vi "Bertta_v09_61.vi"() -> ()   [LabVIEW 2015]
uses:
  x64/Debug/BERTTA.dll
panel:
  out "element":bool
  out "Started:":string
  in  "SHUTDOWN":bool
  in  "MASTER CONTROL":bool
  in  "Tab Control":T1(tab)
  in  "Read Seq":bool
  in  "Save Seq":bool
  in  "Configuration file":path=path "C:/Users/shresplab/Desktop/BerttaConfiguration.lvm" caption="Filename"
  in  "OK Button 2":bool
  out "Boolean":bool
  in  "User (initials)":string
  in  "Project name":string
  in  "Description":string
  out "Output file":string
  out "PUMP1":bool
  out "Target amount":dbl
  out "Scale weight":dbl
  out "Amount now":dbl
  out "Flow rate":dbl
  out "Time to target":dbl format="%<%H:%M:%S>t"
  out "Current step":dbl
  out "Target":dbl
  out "Amount now":dbl
  out "Amount now":dbl
  out "Target":dbl
  out "Current step":dbl
  out "Time to target":dbl format="%<%H:%M:%S>t"
  out "Flow rate":dbl
  out "Amount now":dbl
  out "Scale weight":dbl
  out "Target amount":dbl
  out "PUMP2":bool
  out "Sensor OK 6":bool
  out "Sensor OK 5":bool
  out "Sensor OK 4":bool
  out "Sensor OK 3":bool
  in  "OK Button":bool
  in  "Add comment":string
  out "PUMP3":bool
  out "Target amount":dbl
  out "Scale weight":dbl
  out "Amount now":dbl
  out "Flow rate":dbl
  out "Time to target":dbl format="%<%H:%M:%S>t"
  out "Current step":dbl
  out "Target":dbl
  out "Amount now":dbl
  out "Tr":dbl
  out "Tj in":dbl
  out "Tj out":dbl
  out "T set":dbl
  out "Current step":i32
  out "RPM":dbl
  out "Torque 2":dbl
  out "Waveform Chart 5":dynamicdata(graph)
  out "Waveform Chart 6":dynamicdata(graph)
  out "Waveform Chart 7":dynamicdata(graph)
  in  "Tab Control 2":T2(tab)
  out "Waveform Chart 3":dynamicdata(graph)
  out "Waveform Chart 8":dynamicdata(graph)
  out "Waveform Chart 11":dynamicdata(graph)
  out "Waveform Chart 13":dynamicdata(graph)
  out "Waveform Chart 9":dynamicdata(graph)
  out "Table":string[][](table)=[["14.8.2017 18.06.59", "0,000000", "417,670000", "-0,150000", "1,000000", "22,220000", "23,366837", "23,574959", "23,985852", "23,690000", "240,000000", "4,000000", "0,000000", "397,000000", "-397,000000", "1,000000"], ["14.8.2017 18.07.06", "0,000000", "417,640000", "-0,120000", "1,000000", "22,220000", "23,763115", "23,906257", "23,985694", "23,680000", "240,000000", "4,000000", "0,000000", "397,000000", "-397,000000", "1,000000"], ["14.8.2017 18.07.13", "0,000000", "417,640000", "-0,120000", "1,000000", "22,220000", "23,965922", "24,013440", "23,984906", "23,670000", "240,000000", "4,100000", "3,000000", "397,000000", "-397,000000", "1,000000"], ["14.8.2017 18.07.21", "0,000000", "417,640000", "-0,120000", "1,000000", "22,220000", "23,943860", "23,900110", "23,987113", "23,670000", "240,000000", "4,000000", "0,000000", "397,000000", "-397,000000", "1,000000"], ["14.8.2017 18.07.28", "0,000000", "417,640000", "-0,120000", "1,000000", "22,220000", "23,736328", "23,600018", "23,989004", "23,660000", "240,000000", "4,000000", "0,000000", "397,000000", "-397,000000", "1,000000"], ["14.8.2017 18.07.36", "0,000000", "417,640000", "-0,120000", "1,000000", "22,220000", "23,480910", "23,324538", "23,991053", "23,660000", "240,000000", "4,000000", "0,000000", "397,000000", "-397,000000", "1,000000"], ["14.8.2017 18.07.43", "0,000000", "417,640000", "-0,120000", "2,000000", "22,220000", "23,195579", "23,008270", "23,999093", "23,650000", "240,000000", "4,000000", "0,000000", "397,000000", "-397,000000", "1,000000"], ["14.8.2017 18.07.51", "0,000000", "417,650000", "-417,650000", "1,000000", "22,220000", "22,862541", "22,649021", "24,003979", "23,650000", "240,000000", "4,000000", "0,000000", "397,000000", "-397,000000", "2,000000"], ["14.8.2017 18.07.58", "0,000000", "417,640000", "0,010000", "1,000000", "22,220000", "22,541353", "22,354878", "24,005398", "23,650000", "240,000000", "4,000000", "0,000000", "397,000000", "-397,000000", "1,000000"], ["14.8.2017 18.08.06", "0,000000", "417,640000", "0,010000", "1,000000", "22,220000", "22,347931", "22,253738", "24,007605", "23,640000", "240,000000", "4,100000", "0,000000", "397,000000", "-397,000000", "1,000000"], ["14.8.2017 18.08.13", "0,000000", "417,640000", "0,010000", "1,000000", "22,220000", "22,329030", "22,302102", "24,006028", "23,640000", "240,000000", "4,000000", "0,000000", "395,820000", "-395,820000", "1,000000"], ["14.8.2017 18.08.20", "0,000000", "417,640000", "0,010000", "1,000000", "22,220000", "22,466849", "22,511320", "24,002403", "23,630000", "240,000000", "4,000000", "0,000000", "395,830000", "-0,010000", "1,000000"], ["14.8.2017 18.08.28", "0,000000", "417,640000", "0,010000", "1,000000", "22,220000", "22,707062", "22,835101", "24,000984", "23,620000", "240,000000", "4,000000", "0,000000", "395,830000", "-0,010000", "1,000000"], ["14.8.2017 18.08.35", "0,000000", "417,640000", "0,010000", "1,000000", "22,220000", "23,054104", "23,232979", "24,001299", "23,600000", "240,000000", "4,000000", "0,000000", "395,830000", "-0,010000", "1,000000"], ["14.8.2017 18.08.43", "0,000000", "417,640000", "0,010000", "1,000000", "22,220000", "23,412371", "23,522793", "24,002560", "23,590000", "240,000000", "4,000000", "0,000000", "395,820000", "0,000000", "1,000000"], ["14.8.2017 18.08.51", "0,000000", "417,640000", "0,010000", "1,000000", "22,220000", "23,596247", "23,656125", "24,003821", "23,580000", "240,000000", "4,000000", "0,000000", "395,820000", "0,000000", "1,000000"]]
  in  "Reset":bool
  in  "Numeric 4":dbl=20.0
  in  "Numeric 3":dbl=30.0
  in  "Numeric 2":dbl=40.0
  in  "Numeric 1":dbl=30.0
  in  "Numeric":dbl=20.0
  out "Boolean 12":bool
  out "Boolean 7":bool
  out "Boolean 6":bool
  out "Boolean 5":bool
  out "Boolean 4":bool
  out "Boolean 19":bool
  in  "Numeric 5":dbl=5.0
  in  "Numeric 6":dbl=5.0
  in  "Numeric 7":dbl=5.0
  in  "Numeric 8":dbl=5.0
  in  "T ext / T ext 2":enum32{"External 1", "External 2"}(radio)
  out "Sensor OK":bool
  in  "T fail":dbl=20.0
  in  "?":bool
  in  "T manual setpoint":dbl=20.0
  in  "Lauda port":dbl=9.0
  in  "Manual select":enum32{"Tr", "Tj"}(radio)
  in  "PAUSE":bool
  out "Waveform Chart":dynamicdata(graph)
  out "T external 2":dbl
  out "Led11 5":bool
  in  "Port":i32=10
  in  "Radio Buttons 4":enum32{"Reglo Digital", "Reglo Analog", "PAM"}(radio)
  out "Speed":dbl
  out "mA":dbl format="%#_2g"
  in  "Port":i32=16
  out "RPM":dbl format="%_4f"
  out "Led10 3":bool
  out "Led9 3":bool
  out "Led8 3":bool
  out "Led7 3":bool
  out "Led6 3":bool
  out "Led5 3":bool
  out "Led4 3":bool
  out "Led3 3":bool
  out "Led2 3":bool
  out "Led1 3":bool
  in  "PumpSeq 4":dbl[][](array[numeric])=[[1.0, 1.0, 7.0], [2.0, 1.0, 2.0], [3.0, 1.0, 100.0], [0.0, 0.0, 0.0], [0.0, 0.0, 0.0], [0.0, 0.0, 0.0], [0.0, 0.0, 0.0], [0.0, 0.0, 0.0], [0.0, 0.0, 0.0], [0.0, 0.0, 0.0], [0.0, 1.0, 0.0]]
  in  "?":bool
  out "Flow rate (g/min)":dbl
  out "Scale reading":dbl
  out "Step amount now":dbl
  in  "Grams / min":dbl
  out "Waveform Chart 14":dynamicdata(graph)
  in  "?":bool
  out "Total amount now":dbl
  out "Total time 4":dbl
  out "Total amount target 4":dbl
  out "Led11 4":bool
  in  "Reset 5":bool
  out "Elapsed / step":i32
  out "Time to target":dbl format="%<%H:%M:%S>t"
  out "Led11":bool
  in  "Port":i32=11
  in  "Radio Buttons 2":enum32{"Reglo Digital", "Reglo Analog", "PAM"}(radio)
  out "Speed":dbl
  out "mA":dbl format="%#_2g"
  in  "Port":i32=15
  out "RPM":dbl format="%_4f"
  out "Led10":bool
  out "Led9":bool
  out "Led8":bool
  out "Led7":bool
  out "Led6":bool
  out "Led5":bool
  out "Led4":bool
  out "Led3":bool
  out "Led2":bool
  out "Led1":bool
  in  "PumpSeq 2":dbl[][](array[numeric])=[[1.0, 1.0, 7.0], [2.0, 1.0, 2.0], [3.0, 1.0, 100.0], [0.0, 0.0, 0.0], [0.0, 0.0, 0.0], [0.0, 0.0, 0.0], [0.0, 0.0, 0.0], [0.0, 0.0, 0.0], [0.0, 0.0, 0.0], [0.0, 0.0, 0.0], [0.0, 1.0, 0.0]]
  in  "?":bool
  out "Flow rate (g/min)":dbl
  out "Scale reading":dbl
  out "Step amount now":dbl
  in  "Grams / min":dbl
  out "Waveform Chart 10":dynamicdata(graph)
  in  "?":bool
  out "Total amount now":dbl
  out "Total time 2":dbl
  out "Total amount target 2":dbl
  out "Led11":bool
  in  "Reset 3":bool
  out "Elapsed / step":i32
  out "Time to target":dbl format="%<%H:%M:%S>t"
  out "Led11 3":bool
  in  "Port":i32=12
  in  "Radio Buttons 3":enum32{"Reglo Digital", "Reglo Analog", "PAM"}(radio)
  out "Speed":dbl
  out "mA":dbl format="%#_2g"
  in  "Port":i32=14
  out "RPM":dbl format="%_4f"
  out "Led10 2":bool
  out "Led9 2":bool
  out "Led8 2":bool
  out "Led7 2":bool
  out "Led6 2":bool
  out "Led5 2":bool
  out "Led4 2":bool
  out "Led3 2":bool
  out "Led2 2":bool
  out "Led1 2":bool
  in  "PumpSeq 3":dbl[][](array[numeric])=[[1.0, 1.0, 7.0], [2.0, 1.0, 2.0], [3.0, 1.0, 100.0], [0.0, 0.0, 0.0], [0.0, 0.0, 0.0], [0.0, 0.0, 0.0], [0.0, 0.0, 0.0], [0.0, 0.0, 0.0], [0.0, 0.0, 0.0], [0.0, 0.0, 0.0], [0.0, 1.0, 0.0]]
  in  "?":bool
  out "Flow rate (g/min)":dbl
  out "Scale reading":dbl
  out "Step amount now":dbl
  in  "Grams / min":dbl
  out "Waveform Chart 12":dynamicdata(graph)
  in  "?":bool
  out "Total amount now":dbl
  out "Total time 3":dbl
  out "Total amount target 3":dbl
  out "Led11 2":bool
  in  "Reset 4":bool
  out "Elapsed / step":i32
  out "Time to target":dbl format="%<%H:%M:%S>t"
  in  "Bypass select 2":enum32{"Remote", "Manual"}(radio)=enum."Manual"
  in  "Port":dbl=13.0
  out "RPM":dbl
  out "Torque":dbl
  in  "Set RPM":dbl(slide) scale=0.0..2000.0
  out "Waveform Chart 4":dynamicdata(graph)
  in  "Treshold (T/C)":dbl=0.5
  out "DAQ 9217 (PT100)":errorcluster
  # "Temperature sensor:"
  # "Manual control:"
  # "PUMP & SCALE 1"
  # "STEP"
  # "TOTAL"
  # "PUMP & SCALE 2"
  # "STEP"
  # "TOTAL"
  # "PUMP & SCALE 3"
  # "STEP"
  # "TOTAL"
  # "Manual control"
  # "Secondary temperature sensor"
  # "Device communication"
  # "Temp"
  # "Time"
  # "Grams    /   min"
  # "End of sequence"
  # "Manual control"
  # "Device communication"
  # "Pump configuration"
  # "Scale configuration"
  # "SCALE 1"
  # "Grams    /   min"
  # "End of sequence"
  # "Manual control"
  # "Device communication"
  # "Pump configuration"
  # "Scale configuration"
  # "SCALE 2"
  # "Grams    /   min"
  # "End of sequence"
  # "Manual control"
  # "Device communication"
  # "Pump configuration"
  # "Scale configuration"
  # "SCALE 3"
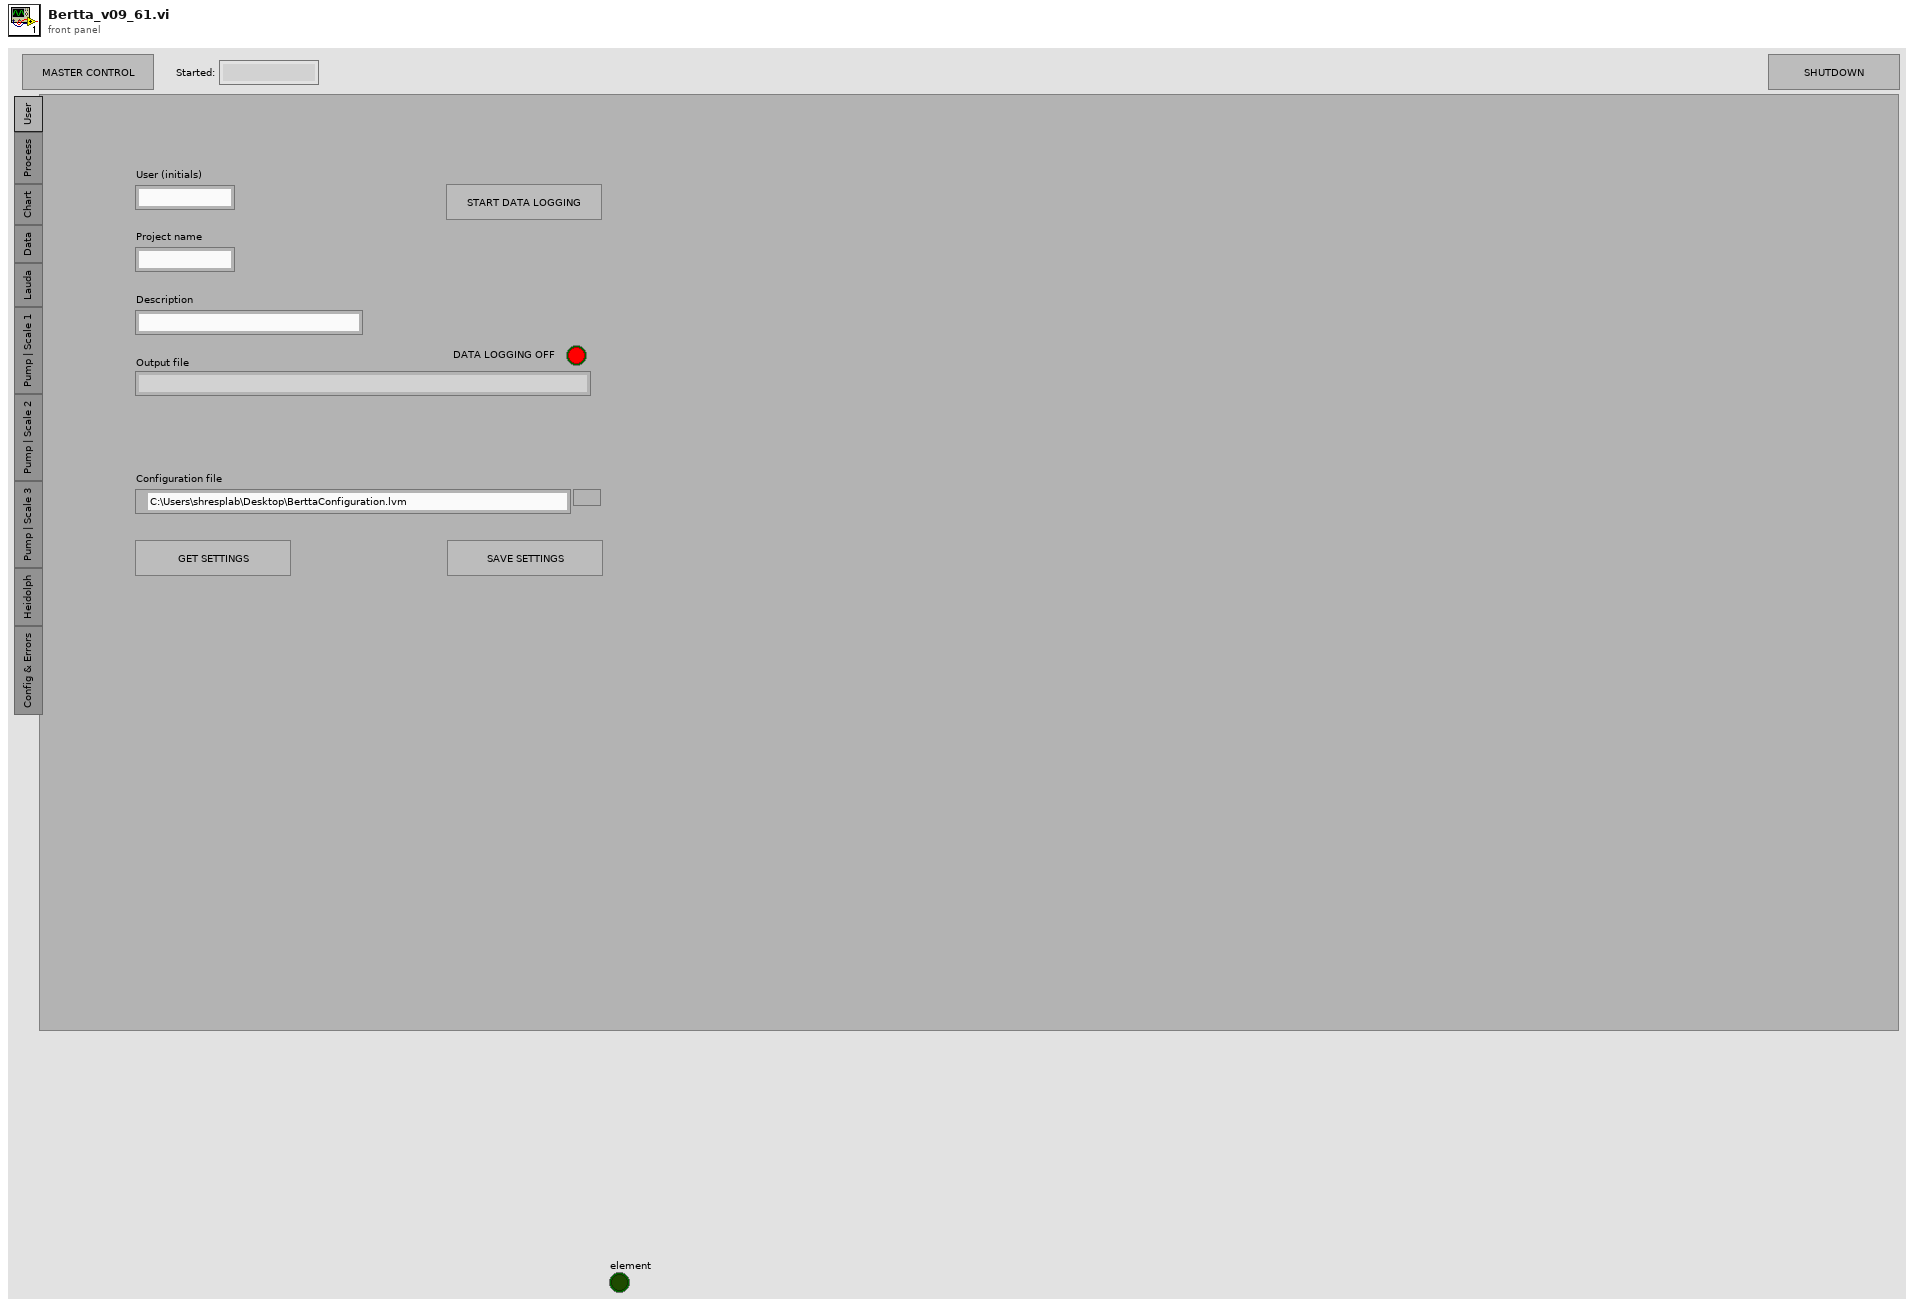
[diagram p1: front panel]
types:
  T1 = enum32{"User", "Process", "Chart", "Data", "Lauda", "Pump | Scale 1", "Pump | Scale 2", "Pump | Scale 3", "Heidolph", "Config & Errors"}
  T2 = enum32{"Temperatures", "Scale / Pump 1", "Scale / Pump 2", "Scale / Pump 3", "RPM / torque"}
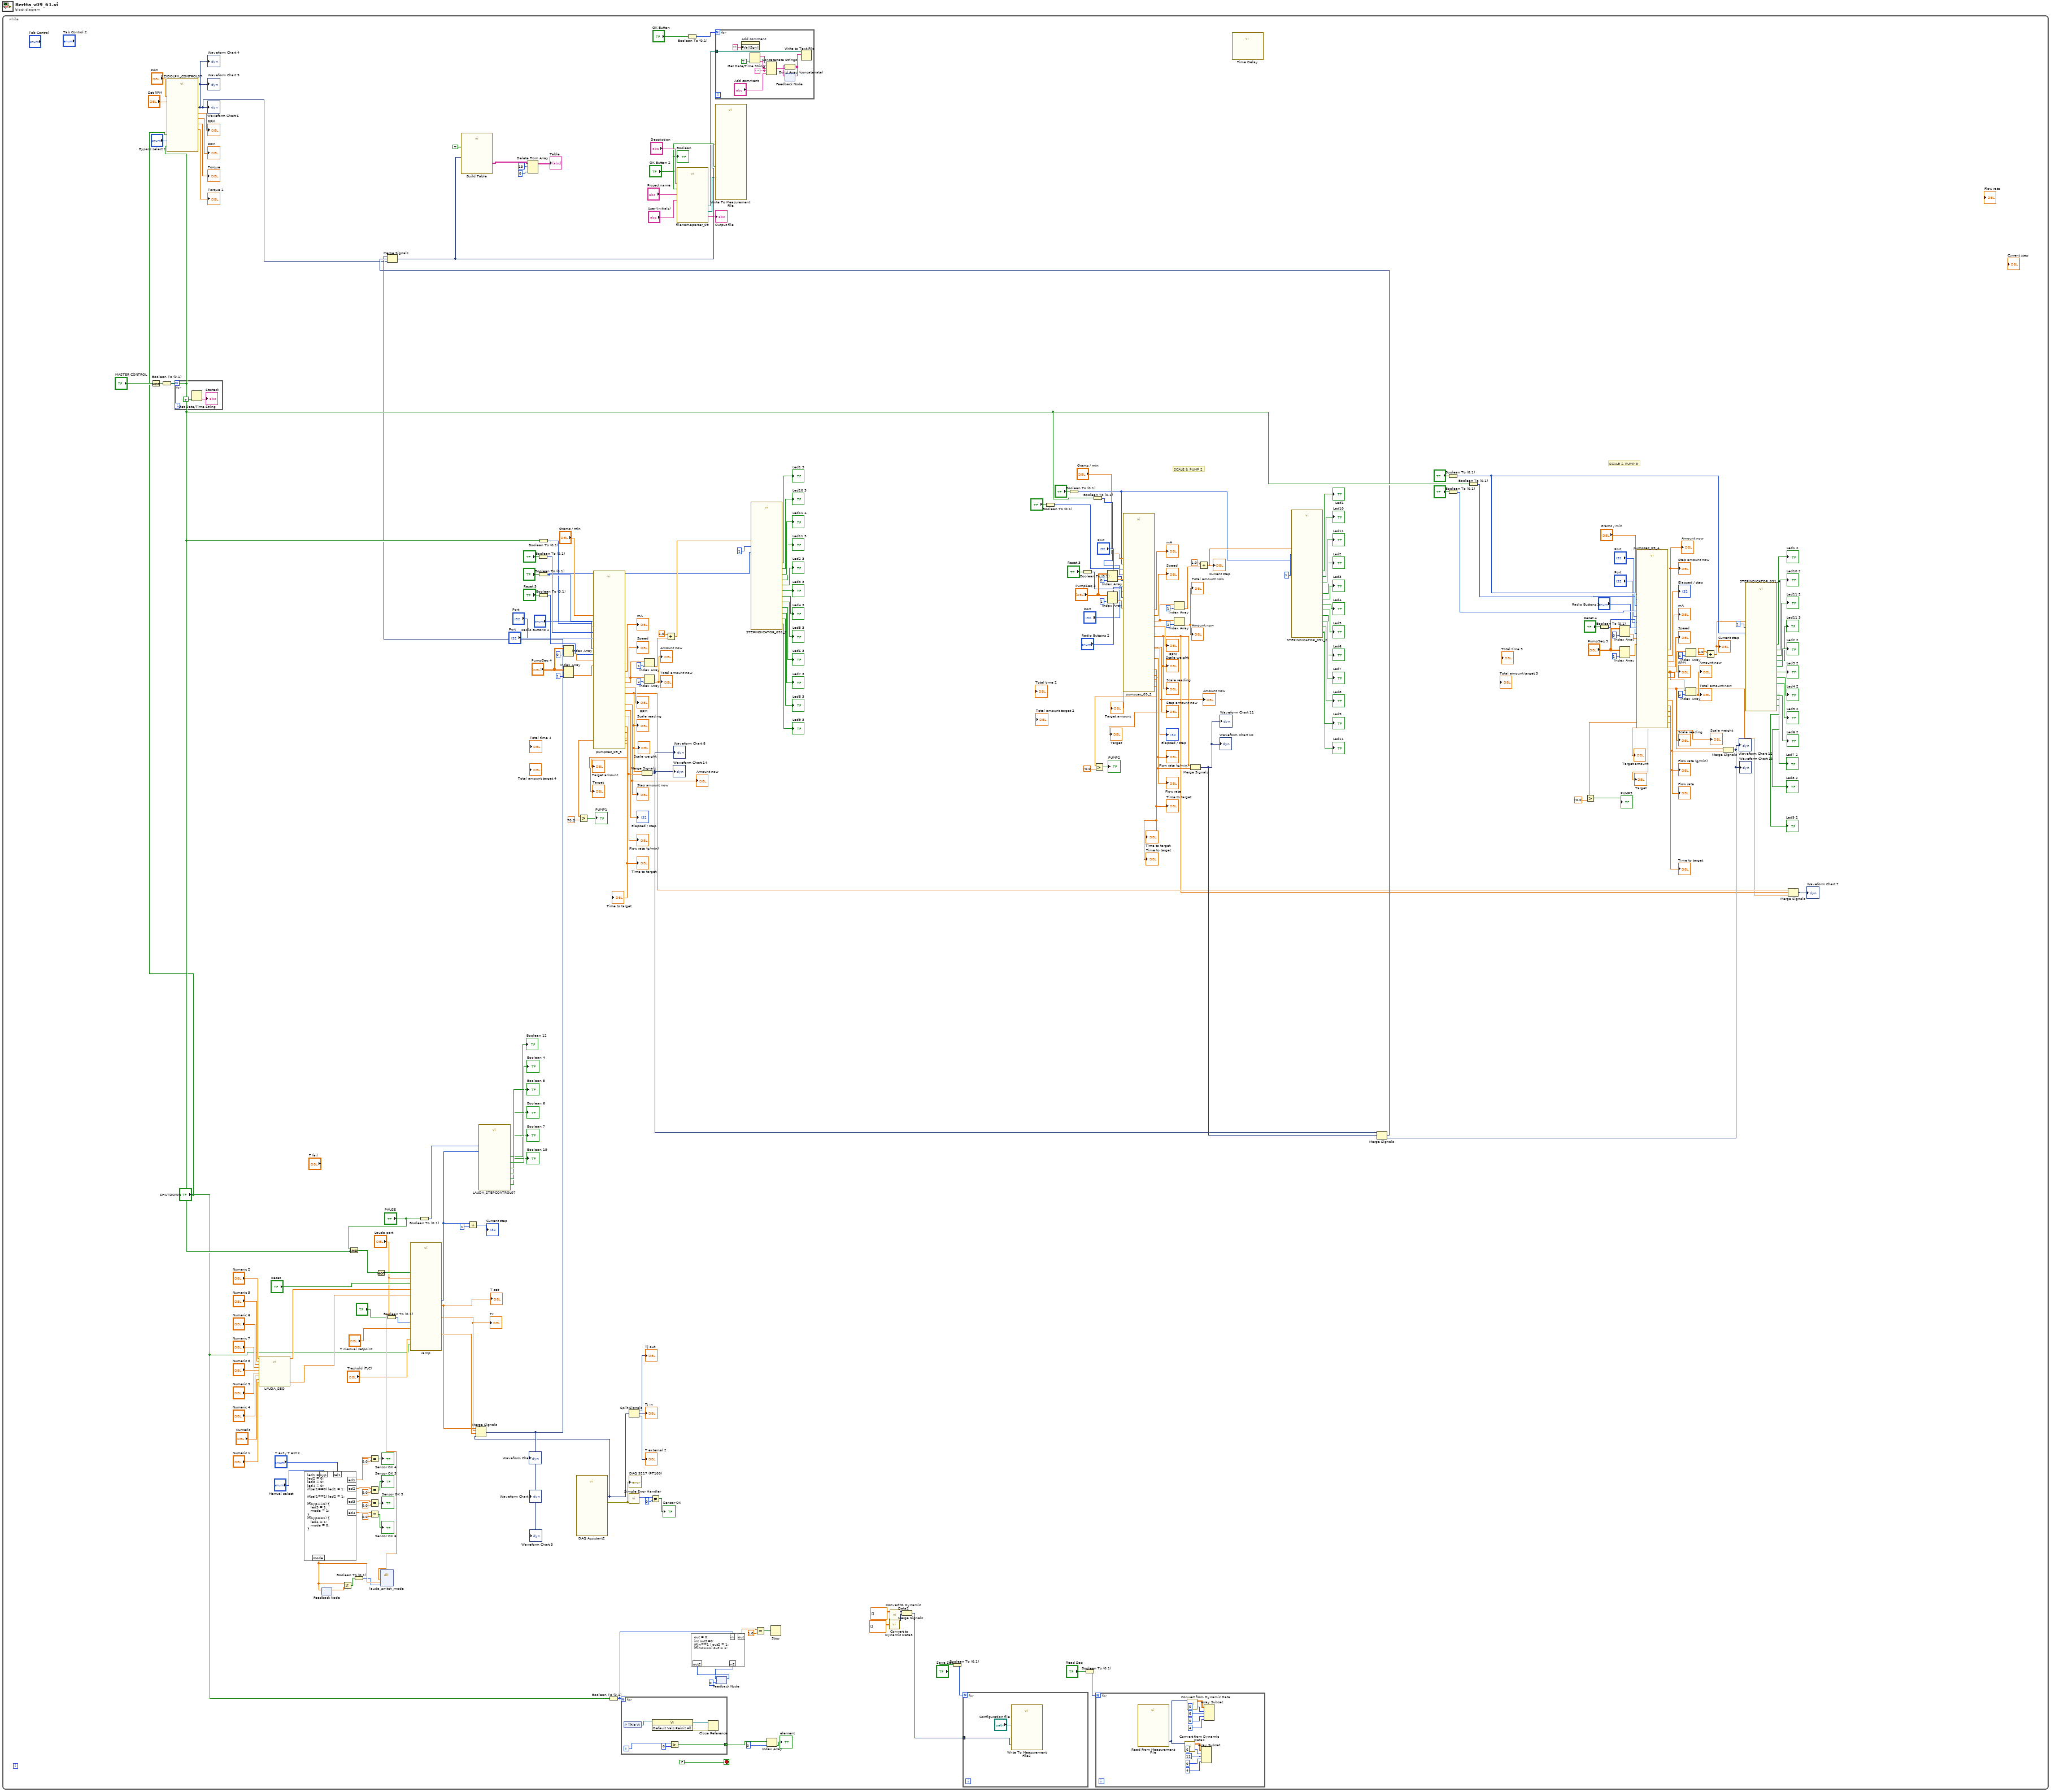
[diagram p0: block diagram]
diagram:
  n1 = while {
    stop <- FALSE stop-if-true
    # "SCALE & PUMP 3"
    # "SCALE & PUMP 2"
    n2 = Not(x="MASTER CONTROL") -> (.not. x?=w239:bool)
    n3 = Boolean To (0,1)(Boolean=w239) -> (0, 1=w240:i16)
    n4 = call "HEIDOLPH_CONTROL07.vi"("master"="MASTER CONTROL", "shutdown"="SHUTDOWN", "Bypass select"="Bypass select 2", "Set RPM"="Set RPM", "Device port"="Port") -> ("Dynamic Data"=w37:dynamicdata, "RPM"=→"RPM":dbl, "RPM 2"=→"RPM":dbl, "Torque"=→"Torque":dbl, "Torque 2"=→"Torque 2":dbl)  [unwired: 2 in]
    "Waveform Chart 4" <- w37
    "Waveform Chart 6" <- w37
    "Waveform Chart 9" <- w37
    n5 = for {
      N: w240 -> [_]
      n6 = Get Date/Time String(want seconds? (F)=TRUE) -> (time string=→"Started:":string)  [unwired: 2 in, 1 out]
    }
    n7 = call "LAUDA_SEQ.vi"("Numeric 2"="Numeric 2", "Numeric 1"="Numeric 1", "Numeric"="Numeric", "Numeric 5"="Numeric 5", "Numeric 6"="Numeric 6", "Numeric 7"="Numeric 7", "Numeric 8"="Numeric 8", "Numeric 3"="Numeric 3", "Numeric 4"="Numeric 4") -> ("output array"=w140:dbl[], "output array 2"=w139:dbl[])  [unwired: 5 in]
    n8 = formula code="led1 = 0;\nled2 = 0;\nled3 = 0;\nled4 = 0;\nif(sel1==0) led1 = 1;\n\nif(sel1==1) led2 = 1;\n\nif(byp==0) {\n   led3 = 1;\n   mode = 1;\n}\nif(byp==1) {\n   led4 = 1;\n   mode = 0;\n}"("sel1"="T ext / T ext 2", "byp"="Manual select") -> ("led1"=w209:dbl, "led2"=w207:dbl, "led3"=w202:dbl, "led4"=w201:dbl, "mode"=w134:dbl)
    n9 = feedback-in #1(w134) -> ()
    n10 = feedback #1() -> (w133:dbl)  [unwired: 1 in]
    n11 = Not Equal?(x=w134, y=w133) -> (x != y?=w131:bool)
    n12 = And(x="PAUSE", y="MASTER CONTROL") -> (x .and. y?=w152:bool)
    n13 = Boolean To (0,1)(Boolean=w131) -> (0, 1=w132:i16)
    n14 = Equal?(x=w209, y=0.0) -> (x = y?=→"Sensor OK 4":bool)
    n15 = Equal?(x=w207, y=0.0) -> (x = y?=→"Sensor OK 3":bool)
    n16 = Equal?(x=w202, y=0.0) -> (x = y?=→"Sensor OK 5":bool)
    n17 = Equal?(x=w201, y=0.0) -> (x = y?=→"Sensor OK 6":bool)
    n18 = Not(x=w152) -> (.not. x?=w151:bool)
    n19 = dll-call lib="C:/Users/shresplab/OneDrive - Kemira Oyj/Documents/Visual Studio 2017/Projects/Bertta/BERTTA/x64/Debug/BERTTA.dll" fn="lauda_switch_mode"("port"="Lauda port", "mode"=w134, "enable"=w132) -> ()  [unwired: 7 in, 2 out]
    n20 = Boolean To (0,1)(Boolean="?") -> (0, 1=w137:i16)
    n21 = call "ramp.vi"("pause"=w151, "manual"=w137, "T_man"="T manual setpoint", "Seq"=w140, "reset"="Reset", "TimeParams"=w139, "shutdown"="SHUTDOWN", "port"="Lauda port", "treshold"="Treshold (T/C)") -> ("T in"=w36:dbl, "STEP"=w3:i32, "T ext"=w21:dbl, "T control"=w22:dbl)  [unwired: 2 in, 1 out]
    "Tr" <- w21
    "T set" <- w22
    n22 = Boolean To (0,1)(Boolean="PAUSE") -> (0, 1=w196:i16)
    n23 = Add(x=w3, y=1) -> (x+y=→"Current step":i32)
    n24 = call "LAUDA_STEPCONTROL07.vi"("step"=w3, "pause"=w196) -> ("Boolean 13"=→"Boolean 19":bool, "Boolean 6"=→"Boolean 6":bool, "Boolean 5"=→"Boolean 5":bool, "Boolean 4"=→"Boolean 4":bool, "Boolean 7"=→"Boolean 7":bool, "Boolean 12"=→"Boolean 12":bool)  [unwired: 4 in]
    n25 = Boolean To (0,1)(Boolean="?") -> (0, 1=w47:i16)
    n26 = Boolean To (0,1)(Boolean="?") -> (0, 1=w57:i16)
    n27 = Boolean To (0,1)(Boolean="MASTER CONTROL") -> (0, 1=w43:i16)
    n28 = Boolean To (0,1)(Boolean="Reset 5") -> (0, 1=w56:i16)
    n29 = Index Array(array="PumpSeq 4", index (col)=0) -> (element=w62:dbl[])  [unwired: 1 in]
    n30 = Index Array(array="PumpSeq 4", index (col)=1) -> (element=w84:dbl[])  [unwired: 1 in]
    n31 = call "DAQ Assistant2"() -> ("data"=w35:dynamicdata, "error out"=w249:errorcluster)  [unwired: 17 in, 1 out]
    "DAQ 9217 (PT100)" <- w249
    n32 = Merge Signals(w22, w21, w36, w35) -> (w38:dynamicdata)
    "Waveform Chart 3" <- w38
    "Waveform Chart" <- w38
    "Waveform Chart 5" <- w38
    n33 = call "pumpsec_09_5.vi"("reset"=w56, "master"=w43, "manual"=w47, "pause"=w57, "Port"="Port", "pump_type"="Radio Buttons 4", "port, Reglo D"="Port", "Target"=w62, "fr_manual"="Grams / min", "Time"=w84) -> ("pumpCtrl"=w16:dbl, "totaltarget"=→"Target":dbl, "target_step"=→"Target amount":dbl, "time_to_target"=→"Time to target" →"Time to target":dbl, "step_fr"=w34:dbl, "amount_step"=→"Amount now" →"Step amount now":dbl, "Reglo D"=→"RPM":dbl, "Scale"=w30:dbl, "mA"=→"mA":dbl, "elapsed_step"=→"Elapsed / step":dbl, "params"=w81:dbl[], "PAM"=→"Speed":dbl)  [unwired: 4 in, 2 out]
    "Scale weight" <- w30
    "Scale reading" <- w30
    "Flow rate (g/min)" <- w34
    n34 = Greater?(x=w16, y=70.0) -> (0:→"PUMP1":bool)
    n35 = Boolean To (0,1)(Boolean="SHUTDOWN") -> (0, 1=w214:i16)
    n36 = for {
      N: w214 -> [_]
      tunnel: [w283] -> w238 mode=indexing
      i -> [w285]
      n37 = control-ref of="This VI"() -> (w288:refnum<vi>)
      n38 = invoke class="VI" method="Default Vals.Reinit All"(reference=w288) -> (reference out=w286:refnum<vi>, error out=w287:errorcluster)  [unwired: 2 in, 1 out]
      n39 = Greater?(x=w285, y=0) -> (0:w283:bool)
      n40 = Close Reference(reference=w286, error in (no error)=w287) -> ()  [unwired: 1 out]
    }
    n41 = Split Signals(w35) -> (→"Tj out":dynamicdata, →"Tj in":dynamicdata, →"T external 2":dynamicdata)  [unwired: 3 in]
    n42 = call <vilib>:"Simple Error Handler.vi"("error in (no error)"=w249) -> ("code out"=w248:i32)  [unwired: 4 in, 4 out]
    n43 = Merge Signals(w30, w34) -> (w41:dynamicdata)
    "Waveform Chart 8" <- w41
    "Waveform Chart 14" <- w41
    n44 = Index Array(array=w81, index=1) -> (element=w78:dbl)
    n45 = Index Array(array=w81, index=2) -> (element=→"Amount now" →"Total amount now":dbl)
    n46 = Not Equal?(x=w248, y=0) -> (x != y?=→"Sensor OK":bool)
    n47 = Add(x=1.0, y=w78) -> (x+y=w77:dbl)
    n48 = call "filenameparser_09.vi"("Description"="Description", "Project name"="Project name", "User (initials)"="User (initials)", "OK Button in"="OK Button 2") -> ("Output file"=→"Output file":string, "appended path 2"=w221:path, "appended path"=w220:path)  [unwired: 5 in]
    n49 = Boolean To (0,1)(Boolean="OK Button") -> (0, 1=w219:i16)
    n50 = for {
      N: w219 -> [_]
      tunnel: w220 -> [w262]
      w266 = " " ("string")
      n51 = property on="Add comment" class="Str"("Val(Sgnl)"="" ("Value (Signaling)")) -> ()  [unwired: 2 in, 2 out]
      n52 = Get Date/Time String(want seconds? (F)=TRUE) -> (date string=w269:string, time string=w267:string)  [unwired: 2 in]
      n53 = Concatenate Strings(w269, w266, w267, w266, "Add comment") -> (w265:string)
      n54 = feedback #2() -> (w264:string[])  [unwired: 1 in]
      n55 = Build Array (concatenate)(w264, w265) -> (w263:string[])
      n56 = feedback-in #2(w263) -> ()
      n57 = Write to Text File(file (use dialog)=w262, text=w263) -> ()  [unwired: 2 in, 3 out]
    }
    n58 = feedback #3(0) -> (w212:i32)
    n59 = formula code="out = 0;\nint out2=0;\nif(in==1 ) out2 = 1;\nif(in2==1) out = 1;"("in"=w214, "in2"=w212) -> ("out"=w216:dbl, "out2"=w213:i32)
    n60 = feedback-in #3(w213) -> ()
    n61 = call "STEPINDICATOR_091_2.vi"("current step"=w77, "enable"=i16 1, "manual"=w47) -> ("Led 8"=→"Led8 3":bool, "Led 10"=→"Led10 3":bool, "Led 11"=→"Led11 4":bool, "Led 7"=→"Led7 3":bool, "Led 1"=→"Led1 3":bool, "Led 6"=→"Led6 3":bool, "Led 2"=→"Led2 3":bool, "Led 12"=→"Led11 5":bool, "Led 5"=→"Led5 3":bool, "Led 4"=→"Led4 3":bool, "Led 3"=→"Led3 3":bool, "Led 9"=→"Led9 3":bool)  [unwired: 1 in]
    n62 = Equal?(x=w216, y=1.0) -> (x = y?=w215:bool)
    n63 = Index Array(array=w238, index=0) -> (element=→"element":bool)
    n64 = Stop(stop? (T)=w215) -> ()
    n65 = call "Convert to Dynamic Data3"("2D Array"=dbl[][] []) -> ("Dynamic Data Type"=w198:dynamicdata)  [unwired: 3 in]
    n66 = call "Convert to Dynamic Data2"("2D Array"=dbl[][] []) -> ("Dynamic Data Type"=w236:dynamicdata)  [unwired: 3 in]
    n67 = Merge Signals(w236, w198) -> (w235:dynamicdata)
    n68 = Boolean To (0,1)(Boolean="Save Seq") -> (0, 1=w234:i16)
    n69 = for {
      N: w234 -> [_]
      tunnel: w235 -> [w282]
      n70 = call "Write To Measurement File2"("Signals"=w282, "Filename"="Configuration file") -> ()  [unwired: 15 in, 3 out]
    }
    n71 = Boolean To (0,1)(Boolean="?") -> (0, 1=w185:i16)
    n72 = Boolean To (0,1)(Boolean="?") -> (0, 1=w126:i16)
    n73 = Boolean To (0,1)(Boolean="Reset 3") -> (0, 1=w182:i16)
    n74 = Boolean To (0,1)(Boolean="Read Seq") -> (0, 1=w231:i16)
    n75 = Boolean To (0,1)(Boolean="MASTER CONTROL") -> (0, 1=w176:i16)
    n76 = for {
      N: w231 -> [_]
      n77 = call "Read From Measurement File"() -> ("Signals"=w271:dynamicdata)  [unwired: 6 in, 5 out]
      n78 = call "Convert from Dynamic Data2"("Dynamic Data Type"=w271) -> ("Array"=w270:dbl[][])  [unwired: 3 in]
      n79 = call "Convert from Dynamic Data"("Dynamic Data Type"=w271) -> ("Array"=w278:dbl[][])  [unwired: 3 in]
      n80 = Array Subset(array=w270, index (row)=6 ("index"), length (row)=11 ("length"), index (col)=0 ("index"), length (col)=4 ("length")) -> ()  [unwired: 1 out]
      n81 = Array Subset(array=w278, index (row)=0 ("index"), length (row)=6 ("length"), index (col)=0 ("index"), length (col)=4 ("length")) -> ()  [unwired: 1 out]
    }
    n82 = Index Array(array="PumpSeq 2", index (col)=0 ("disabled index (col)")) -> (element=w188:dbl[])  [unwired: 1 in]
    n83 = Index Array(array="PumpSeq 2", index (col)=1 ("disabled index (col)")) -> (element=w187:dbl[])  [unwired: 1 in]
    n84 = call "pumpsec_09_2.vi"("reset"=w182, "master"=w176, "manual"=w126, "pause"=w185, "Port"="Port", "pump_type"="Radio Buttons 2", "port, Reglo D"="Port", "Target"=w188, "fr_manual"="Grams / min", "Time"=w187) -> ("pumpCtrl"=w12:dbl, "totaltarget"=→"Target":dbl, "target_step"=→"Target amount":dbl, "time_to_target"=→"Time to target" →"Time to target" →"Time to target":dbl, "step_fr"=w33:dbl, "amount_step"=→"Amount now" →"Step amount now":dbl, "Reglo D"=→"RPM":dbl, "Scale"=w29:dbl, "mA"=→"mA":dbl, "elapsed_step"=→"Elapsed / step":dbl, "params"=w177:dbl[], "PAM"=→"Speed":dbl)  [unwired: 4 in, 2 out]
    "Scale weight" <- w29
    "Flow rate" <- w33
    "Scale reading" <- w29
    "Flow rate (g/min)" <- w33
    n85 = Greater?(x=w12, y=70.0) -> (0:→"PUMP2":bool)
    n86 = Index Array(array=w177, index=1) -> (element=w180:dbl)
    n87 = Index Array(array=w177, index=2) -> (element=→"Amount now" →"Total amount now":dbl)
    n88 = Merge Signals(w29, w33) -> (w44:dynamicdata)
    "Waveform Chart 11" <- w44
    "Waveform Chart 10" <- w44
    n89 = Add(x=1.0, y=w180) -> (x+y=w170:dbl)
    "Current step" <- w170
    n90 = call "Time Delay"() -> ()  [unwired: 11 in, 1 out]
    n91 = call "STEPINDICATOR_091_2.vi"("current step"=w170, "enable"=i16 1, "manual"=w126) -> ("Led 8"=→"Led8":bool, "Led 10"=→"Led10":bool, "Led 11"=→"Led11":bool, "Led 7"=→"Led7":bool, "Led 1"=→"Led1":bool, "Led 6"=→"Led6":bool, "Led 2"=→"Led2":bool, "Led 12"=→"Led11":bool, "Led 5"=→"Led5":bool, "Led 4"=→"Led4":bool, "Led 3"=→"Led3":bool, "Led 9"=→"Led9":bool)  [unwired: 1 in]
    n92 = Boolean To (0,1)(Boolean="?") -> (0, 1=w120:i16)
    n93 = Boolean To (0,1)(Boolean="?") -> (0, 1=w119:i16)
    n94 = Boolean To (0,1)(Boolean="MASTER CONTROL") -> (0, 1=w121:i16)
    n95 = Boolean To (0,1)(Boolean="Reset 4") -> (0, 1=w99:i16)
    n96 = Index Array(array="PumpSeq 3", index (col)=0 ("disabled index (col)")) -> (element=w103:dbl[])  [unwired: 1 in]
    n97 = Index Array(array="PumpSeq 3", index (col)=1 ("disabled index (col)")) -> (element=w102:dbl[])  [unwired: 1 in]
    n98 = call "pumpsec_09_4.vi"("reset"=w99, "master"=w121, "manual"=w120, "pause"=w119, "Port"="Port", "pump_type"="Radio Buttons 3", "port, Reglo D"="Port", "Target"=w103, "fr_manual"="Grams / min", "Time"=w102) -> ("pumpCtrl"=w9:dbl, "totaltarget"=→"Target":dbl, "target_step"=→"Target amount":dbl, "time_to_target"=→"Time to target":dbl, "step_fr"=w32:dbl, "amount_step"=→"Amount now" →"Step amount now":dbl, "Reglo D"=→"RPM":dbl, "Scale"=w28:dbl, "mA"=→"mA":dbl, "elapsed_step"=→"Elapsed / step":dbl, "params"=w86:dbl[], "PAM"=→"Speed":dbl)  [unwired: 4 in, 2 out]
    "Scale weight" <- w28
    "Flow rate" <- w32
    "Scale reading" <- w28
    "Flow rate (g/min)" <- w32
    n99 = Greater?(x=w9, y=70.0) -> (0:→"PUMP3":bool)
    n100 = Index Array(array=w86, index=1) -> (element=w87:dbl)
    n101 = Index Array(array=w86, index=2) -> (element=→"Amount now" →"Total amount now":dbl)
    n102 = Add(x=1.0, y=w87) -> (x+y=w85:dbl)
    "Current step" <- w85
    n103 = Merge Signals(w28, w32) -> (w40:dynamicdata)
    "Waveform Chart 13" <- w40
    "Waveform Chart 12" <- w40
    n104 = Merge Signals(w41, w44, w40) -> (w39:dynamicdata)
    n105 = Merge Signals(w38, w39, w37) -> (w226:dynamicdata)
    n106 = call "Build Table"("Include time data"=TRUE, "Signals"=w226) -> ("Table"=w225:string[][])  [unwired: 3 in, 6 out]
    n107 = Delete From Array(array=w225, length=13, index (col)=0 ("index (row)")) -> (array with subset deleted=→"Table":string[][])  [unwired: 1 in, 1 out]
    n108 = call "Write To Measurement File"("Signals"=w226, "Enable"="OK Button 2", "Filename"=w221) -> ()  [unwired: 14 in, 3 out]
    n109 = call "STEPINDICATOR_091_4.vi"("current step"=w85, "enable"=i16 1, "manual"=w120) -> ("Led 8"=→"Led8 2":bool, "Led 10"=→"Led10 2":bool, "Led 11"=→"Led11 2":bool, "Led 7"=→"Led7 2":bool, "Led 1"=→"Led1 2":bool, "Led 6"=→"Led6 2":bool, "Led 2"=→"Led2 2":bool, "Led 12"=→"Led11 3":bool, "Led 5"=→"Led5 2":bool, "Led 4"=→"Led4 2":bool, "Led 3"=→"Led3 2":bool, "Led 9"=→"Led9 2":bool)  [unwired: 1 in]
    n110 = Merge Signals(w30, w29, w28) -> (→"Waveform Chart 7":dynamicdata)
    "Boolean" <- "OK Button 2"
  }
